vi "Viavi - openRefs.vi"(8 "error in (no error)":errorcluster {"code" format="Error %.0f"}, 11 "Viavi - strictRefs In":T1) -> (0 "error out":errorcluster {"code" format="Error %.0f"}, 2 "GObjectsFound":i32, 3 "Viavi - strictRefs Out":T1, 4 "FPObjectsLabels":string[](array[string]))   [LabVIEW 2017]
doc: "This VI opens the calling (or parent) VIs FP control, pane, and spitter refnums programatically and builds them into a cluster of GObject Refnums."
uses:
  Controls/Viavi - objectRefs.ctl
  <vilib>/Utility/error.llb/Error Cluster From Error Code.vi
  <vilib>/ErrorRing/Error Ring.xnode
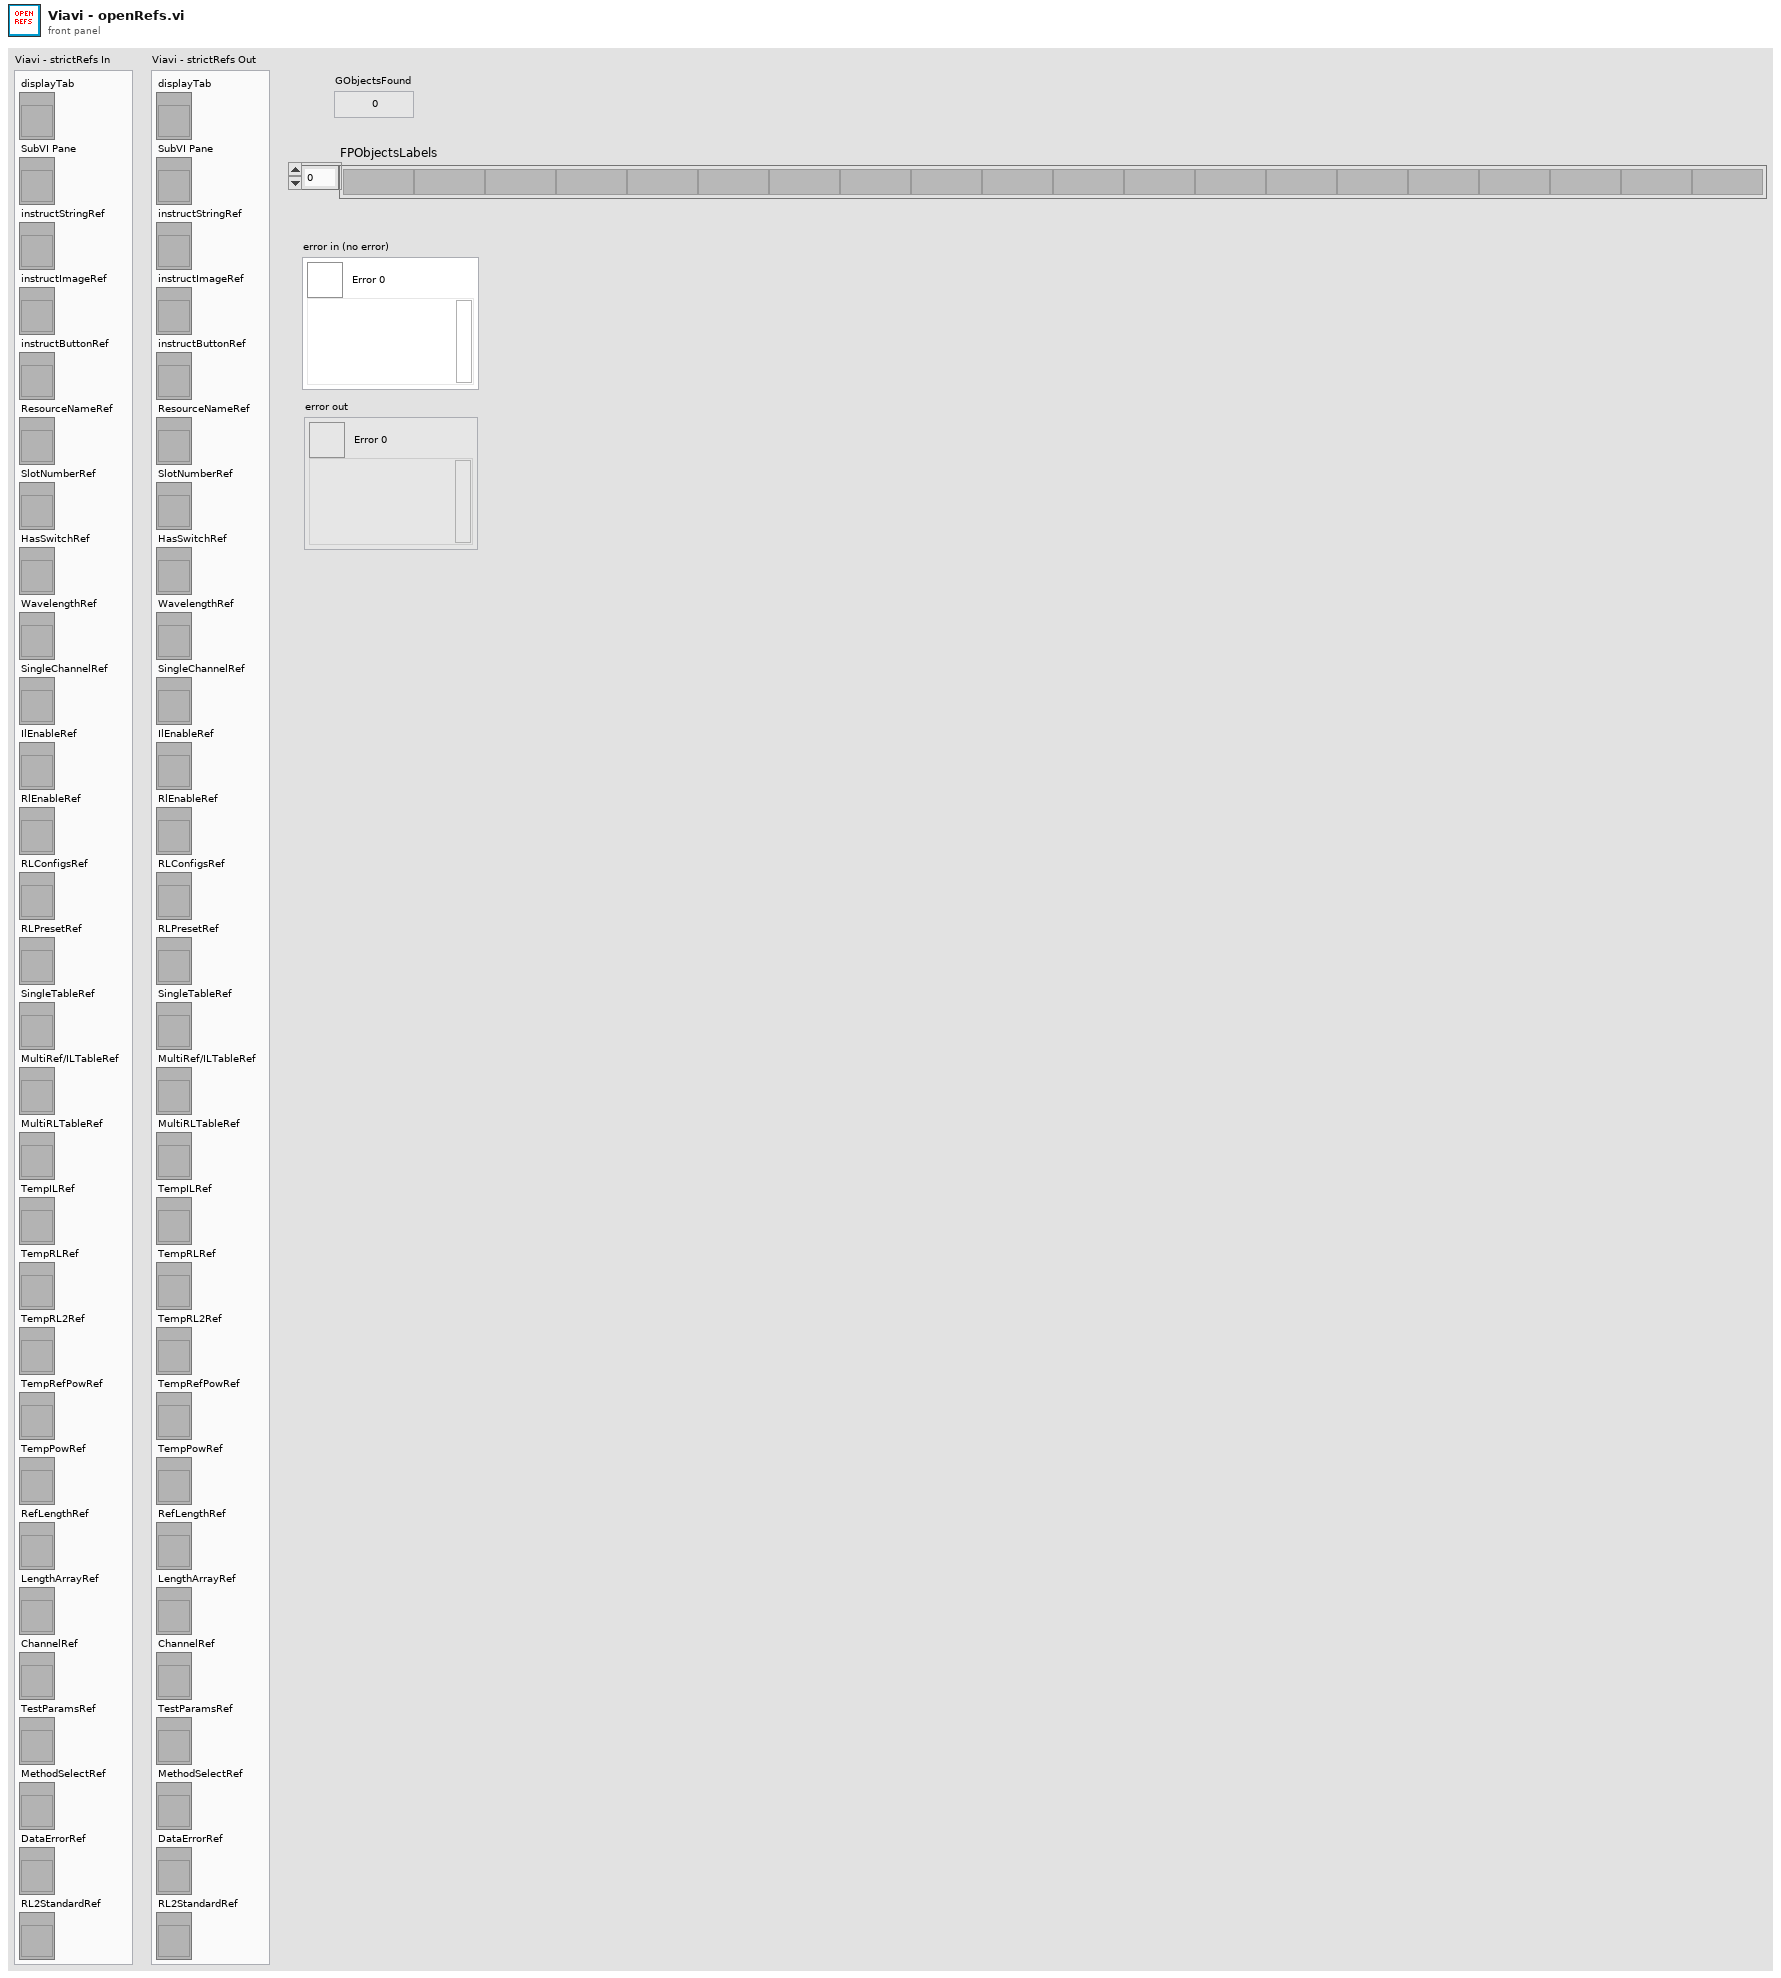
[diagram p1: front panel]
types:
  T1 = typedef "Viavi - objectRefs.ctl" = cluster{"displayTab":refnum<vi>, "SubVI Pane":refnum<vi>, "instructStringRef":refnum<vi>, "instructImageRef":refnum<vi>, "instructButtonRef":refnum<vi>, "ResourceNameRef":refnum<vi>, "SlotNumberRef":refnum<vi>, "HasSwitchRef":refnum<vi>, "WavelengthRef":refnum<vi>, "SingleChannelRef":refnum<vi>, "IlEnableRef":refnum<vi>, "RlEnableRef":refnum<vi>, "RLConfigsRef":refnum<vi>, "RLPresetRef":refnum<vi>, "SingleTableRef":refnum<vi>, "MultiRef/ILTableRef":refnum<vi>, "MultiRLTableRef":refnum<vi>, "TempILRef":refnum<vi>, "TempRLRef":refnum<vi>, "TempRL2Ref":refnum<vi>, "TempRefPowRef":refnum<vi>, "TempPowRef":refnum<vi>, "RefLengthRef":refnum<vi>, "LengthArrayRef":refnum<vi>, "ChannelRef":refnum<vi>, "TestParamsRef":refnum<vi>, "MethodSelectRef":refnum<vi>, "DataErrorRef":refnum<vi>, "RL2StandardRef":refnum<vi>}
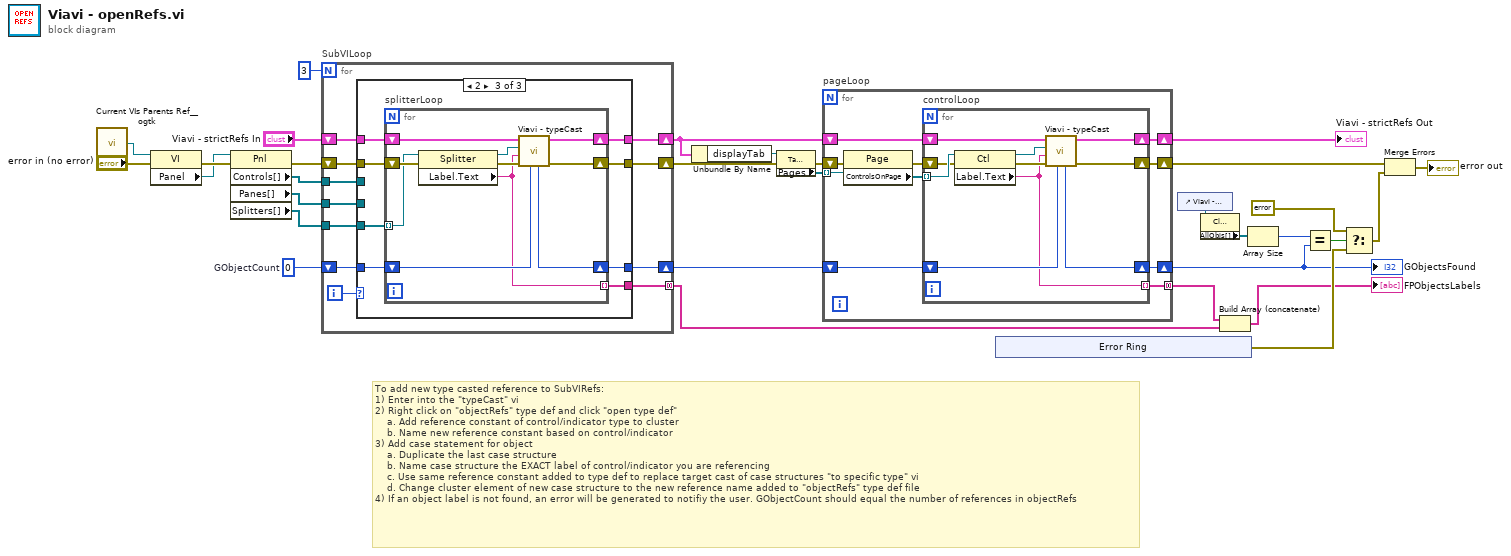
[diagram p0: block diagram]
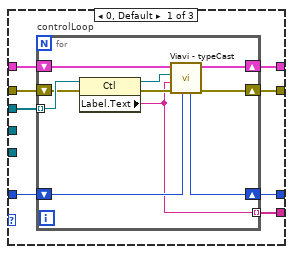
[diagram p2: hidden frame]
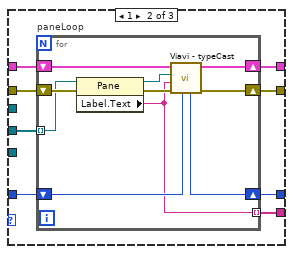
[diagram p3: hidden frame]
diagram:
  w23 = 0  # GObjectCount
  # "To add new type casted reference to SubVIRefs:\n1) Enter into the \"typeCast\" vi\n2) Right click on \"objectRefs\" type def and click \"open type def\"\n    a. Add reference constant of control/indicator type to cluster\n    b. Name new reference constant based on control/indicator\n3) Add case statement for object\n    a. Duplicate the last case structure\n    b. Name case structure the EXACT label of control/indicator you are referencing\n    c. Use same reference constant added to type def to replace target cast of case structures \"to specific type\" vi\n    d. Change cluster element of new case structure to the new reference name added to \"objectRefs\" type def file\n4) If an object label is not found, an error will be generated to notifiy the user. GObjectCount should equal the number of references in objectRefs"
  n1 = call <userlib>:"Current VIs Parents Ref__ogtk.vi"() -> ("Calling VI's Reference"=w17:refnum<vi>)  [unwired: 2 in]
  n2 = property class="VI"(reference=w17, error in="error in (no error)") -> (error out=w30:errorcluster, "Panel"=w28:refnum<vi>)  [unwired: 1 out]
  n3 = property class="Pnl"(reference=w28, error in=w30) -> (error out=w29:errorcluster, "Controls[]"=w24:refnum<vi>[], "Panes[]"=w26:refnum<vi>[], "Splitters[]"=w25:refnum<vi>[])  [unwired: 1 out]
  n4 = for "SubVILoop" {
    N: 3 -> [_]
    tunnel: w24 -> [w42]
    shift-right: [w40] -> w14
    shift-left: w29 -> [w41]
    shift-right: [w38] -> w11
    shift-left: "Viavi - strictRefs In" -> [w39]
    tunnel: w26 -> [w36]
    tunnel: w25 -> [w35]
    shift-right: [w33] -> w10
    shift-left: w23 -> [w34]
    tunnel: [w32] -> w9 mode=concatenating
    i -> [w37]
    n5 = case shown="2" w37 {
      tunnel: w42 -> [w50 _ _]
      tunnel: w41 -> [w49 w68 w86]
      tunnel: [w48 w67 w85] -> w40
      tunnel: w39 -> [w47 w66 w84]
      tunnel: [w46 w65 w83] -> w38
      tunnel: w36 -> [_ w61 _]
      tunnel: w35 -> [_ _ w79]
      tunnel: w34 -> [w44 w63 w81]
      tunnel: [w45 w64 w82] -> w33
      tunnel: [w43 w62 w80] -> w32
      frame 0, Default {
        n6 = for "controlLoop" {
          tunnel: w50 -> [w60] mode=indexing
          shift-right: [w54] -> w48
          shift-left: w49 -> [w59]
          shift-right: [w55] -> w46
          shift-left: w47 -> [w58]
          shift-right: [w52] -> w45
          shift-left: w44 -> [w53]
          tunnel: [w51] -> w43 mode=indexing
          n7 = property class="Ctl"(reference=w60, error in=w59) -> (reference out=w57:refnum<vi>, error out=w56:errorcluster, "Label.Text"=w51:string)
          n8 = call "Viavi - typeCast.vi"("Ref Count In"=w53, "error in"=w56, "Label Name"=w51, "Input Refnum"=w57, "Viavi - strictRefs In"=w58) -> ("error out"=w54:errorcluster, "Viavi - strictRefs Out"=w55:T1, "Ref Count Out"=w52:i32)  [unwired: 3 in, 1 out]
        }
      }
      frame 1 {
        n9 = for "paneLoop" {
          shift-right: [w73] -> w67
          shift-left: w68 -> [w78]
          shift-right: [w74] -> w65
          shift-left: w66 -> [w77]
          shift-right: [w71] -> w64
          shift-left: w63 -> [w72]
          tunnel: [w70] -> w62 mode=indexing
          tunnel: w61 -> [w69] mode=indexing
          n10 = property class="Pane"(reference=w69, error in=w78) -> (reference out=w76:refnum<vi>, error out=w75:errorcluster, "Label.Text"=w70:string)
          n11 = call "Viavi - typeCast.vi"("Ref Count In"=w72, "error in"=w75, "Label Name"=w70, "Input Refnum"=w76, "Viavi - strictRefs In"=w77) -> ("error out"=w73:errorcluster, "Viavi - strictRefs Out"=w74:T1, "Ref Count Out"=w71:i32)  [unwired: 3 in, 1 out]
        }
      }
      frame 2 {
        n12 = for "splitterLoop" {
          shift-right: [w91] -> w85
          shift-left: w86 -> [w96]
          shift-right: [w92] -> w83
          shift-left: w84 -> [w95]
          shift-right: [w89] -> w82
          shift-left: w81 -> [w90]
          tunnel: [w88] -> w80 mode=indexing
          tunnel: w79 -> [w87] mode=indexing
          n13 = property class="Splitter"(reference=w87, error in=w96) -> (reference out=w94:refnum<vi>, error out=w93:errorcluster, "Label.Text"=w88:string)
          n14 = call "Viavi - typeCast.vi"("Ref Count In"=w90, "error in"=w93, "Label Name"=w88, "Input Refnum"=w94, "Viavi - strictRefs In"=w95) -> ("error out"=w91:errorcluster, "Viavi - strictRefs Out"=w92:T1, "Ref Count Out"=w89:i32)  [unwired: 3 in, 1 out]
        }
      }
    }
  }
  n15 = Unbundle By Name(w11) -> ("displayTab"=w15:refnum<vi>)
  n16 = property class="TabCtl (strict)"(reference=w15, error in=w14) -> (error out=w12:errorcluster, "Pages"=w13:refnum<vi>[])  [unwired: 1 out]
  n17 = for "pageLoop" {
    tunnel: w13 -> [w105] mode=indexing
    shift-right: [w100] -> w7
    shift-left: w10 -> [w101]
    tunnel: [w99] -> w8 mode=concatenating
    shift-right: [w98] -> w2
    shift-left: w12 -> [w106]
    shift-right: [w97] -> w3
    shift-left: w11 -> [w102]
    n18 = property class="Page"(reference=w105, error in=w106) -> (error out=w104:errorcluster, "ControlsOnPage"=w103:refnum<vi>[])  [unwired: 1 out]
    n19 = for "controlLoop" {
      tunnel: w103 -> [w116] mode=indexing
      shift-right: [w110] -> w98
      shift-left: w104 -> [w115]
      shift-right: [w111] -> w97
      shift-left: w102 -> [w114]
      shift-right: [w108] -> w100
      shift-left: w101 -> [w109]
      tunnel: [w107] -> w99 mode=indexing
      n20 = property class="Ctl"(reference=w116, error in=w115) -> (reference out=w113:refnum<vi>, error out=w112:errorcluster, "Label.Text"=w107:string)
      n21 = call "Viavi - typeCast.vi"("Ref Count In"=w109, "error in"=w112, "Label Name"=w107, "Input Refnum"=w113, "Viavi - strictRefs In"=w114) -> ("error out"=w110:errorcluster, "Viavi - strictRefs Out"=w111:T1, "Ref Count Out"=w108:i32)  [unwired: 3 in, 1 out]
    }
  }
  "GObjectsFound" <- w7
  "Viavi - strictRefs Out" <- w3
  n22 = xnode "Error Ring"() -> ("error out"=w19:errorcluster)
  n23 = control-ref of="Viavi - strictRefs In"() -> (w6:refnum<vi>)
  n24 = property class="Clust (strict)"(reference=w6) -> ("AllObjs[]"=w5:refnum<vi>[])  [unwired: 1 in, 2 out]
  n25 = Build Array (concatenate)(w8, w9) -> (→"FPObjectsLabels":string[])
  n26 = Array Size(array=w5) -> (size(s)=w4:i32)
  n27 = Equal?(x=w4, y=w7) -> (x = y?=w22:bool)
  n28 = Select(t=errorcluster {"status"=FALSE, "code"=0, "source"=""} ("error in (no error)"), s=w22, f=w19) -> (s? t:f=w20:errorcluster)
  n29 = Merge Errors(w2, w20) -> (→"error out":errorcluster)
